vi "niRFUtil MASMT Resample (constant to constant)_Resample (MultiCh, SGL).vi"(4 "max decimation":i32=1000, 6 "Resample FIR":sgl[](array[numeric]), 7 "reset?":bool, 8 "error in (no error)":errorcluster, 9 "config":T1 {"timing jitter" items=["Interpolation", "Rounding"]}, 10 "anti-aliasing?":bool=TRUE, 11 "X":sgl[][](array[numeric])) -> (0 "error out":errorcluster, 2 "t0":sgl, 3 "Y":sgl[][](array[numeric]))   [LabVIEW 2015, in "niRFUtil.lvlib"]
uses:
  niRFUtil.lvlib
  Utilities/niRFMASMT_FFT.dll
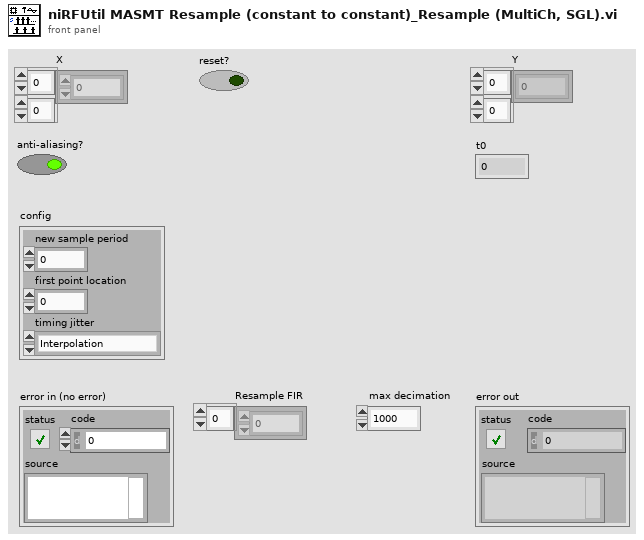
[diagram p1: front panel]
types:
  T1 = cluster{"new sample period":sgl, "first point location":sgl, "timing jitter":i32}
  T2 = cluster{"preConditionLen":i32, "extractFilterLeftLen":i32, "extractFilterRightLen":i32, "extractFilterMethod":i32, "extractFilterScaling":dbl, "samplingPeriod":dbl, "startTime":dbl, "offset":dbl, "index":i32}
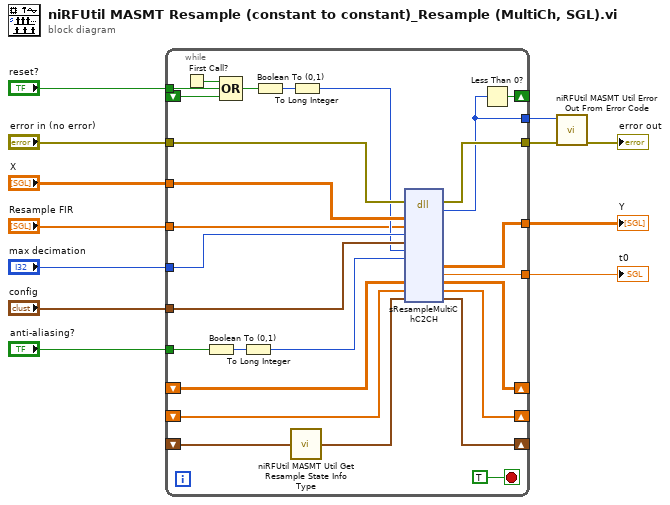
[diagram p0: block diagram]
diagram:
  n1 = while {
    tunnel: "X" -> [w39]
    tunnel: "config" -> [w38]
    tunnel: "error in (no error)" -> [w37]
    tunnel: [w36] -> w1
    tunnel: "anti-aliasing?" -> [w35]
    tunnel: "Resample FIR" -> [w14]
    tunnel: "max decimation" -> [w33]
    tunnel: [w22] -> w12
    tunnel: [w31] -> w11
    tunnel: [w30] -> w2
    tunnel: "reset?" -> [w20]
    shift-right: [w27] -> _
    shift-left: _ -> [w13]
    shift-right: [w28] -> _
    shift-left: _ -> [w24]
    shift-right: [w21] -> _
    shift-left: _ -> [w19]
    shift-right: [w26] -> _
    shift-left: _ -> [w15]
    stop <- TRUE stop-if-true
    n2 = First Call?() -> (First Call?: T/F=w16:bool)
    n3 = Boolean To (0,1)(Boolean=w35) -> (0, 1=w34:i16)
    n4 = Compound Arithmetic op=OR(w16, w20, w19) -> (w17:bool)
    n5 = To Long Integer(number=w34) -> (32bit integer=w32:i32)
    n6 = Boolean To (0,1)(Boolean=w17) -> (0, 1=w18:i16)
    n7 = call "niRFUtil MASMT Util Get Resample State Info Type.vi"("resample state info in"=w24) -> ("resample state info out"=w23:T2)
    n8 = To Long Integer(number=w18) -> (32bit integer=w29:i32)
    n9 = dll-call lib="C:/Perforce/semoore-sales/Customers/NATI-3813/Noise Floor/LV Filters/ParallelComplexFilterRFUtil/niRFUtil/MASMT/Utilities/niRFMASMT_FFT.*" fn="sResampleMultiChC2CH"(error in=w37, "xH"=w39, "pfilterCoefH"=w14, "pfilterMaxDecimation"=w33, "config"=w38, "reset"=w29, "bandLimit"=w32, "xBufferH"=w13, "extractFilterH"=w15, "state"=w23) -> (error out=w31:errorcluster, "error"=w22:i32, "yH"=w30:sgl[][], "t0"=w36:sgl, "xBufferH"=w27:sgl[][], "extractFilterH"=w26:sgl[], "state"=w28:T2)  [unwired: 10 in, 1 out]
    n10 = Less Than 0?(x=w22) -> (x < 0?=w21:bool)
  }
  "t0" <- w1
  "Y" <- w2
  n11 = call "niRFUtil MASMT Util Error Out From Error Code.vi"("error in (no error)"=w11, "error code"=w12) -> ("error out"=→"error out":errorcluster)  [unwired: 9 in]
